vi "保存生产数据.vi"(2 "输入簇":cluster{"载具码":string, "产品码":string, "线号显示":i32}) -> (0 "error out":errorcluster caption="错误输出")   [LabVIEW 2014]
uses:
  Global.vi
  <vilib>/Utility/config.llb/Write Key (Double).vi
  <vilib>/Utility/config.llb/Write Key (String).vi
  <vilib>/Utility/config.llb/NI_LVConfig.lvlib
panel:
  out "File out":path
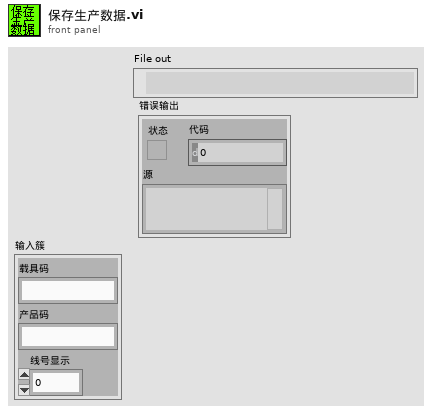
[diagram p1: front panel]
types:
  T1 = typedef "NI_LVConfig.lvlib/Config Data RefNum.ctl" = refnum<k1>
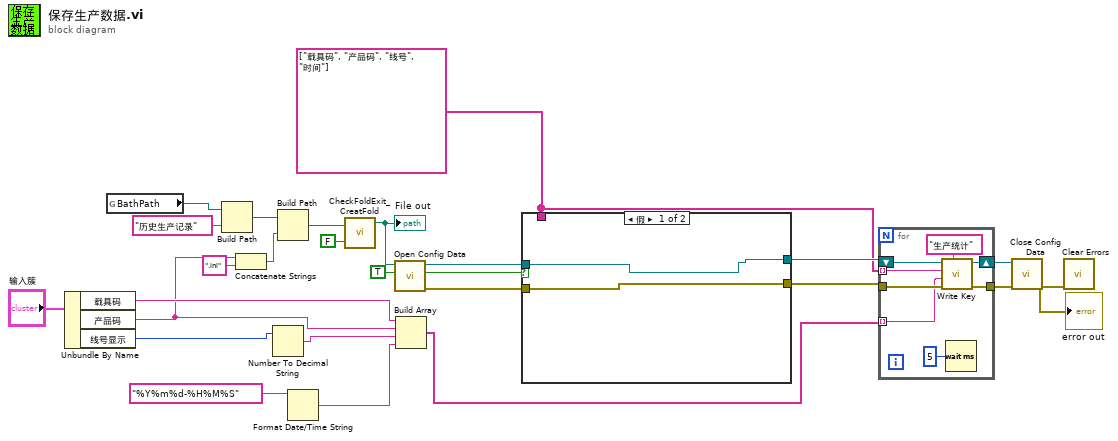
[diagram p0: block diagram]
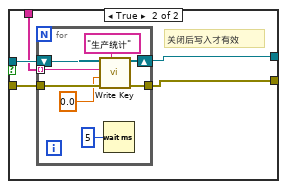
[diagram p2: hidden frame]
diagram:
  w7 = string[] ["载具码", "产品码", "线号", "时间"]
  n1 = Unbundle By Name("输入簇") -> ("载具码"=w10:string, "产品码"=w3:string, "线号显示"=w9:i32)
  n2 = global read "Global.vi" "BathPath"() -> (w21:path)
  n3 = Build Path(base path=w21, name or relative path="历史生产记录" ("名称或相对路径")) -> (appended path=w20:path)
  n4 = Concatenate Strings(w3, ".ini" ("字符串")) -> (w2:string)
  n5 = Number To Decimal String(number=w9) -> (decimal integer string=w8:string)  [unwired: 1 in]
  n6 = Build Path(base path=w20, name or relative path=w2) -> (appended path=w19:path)
  n7 = Format Date/Time String(time format string (%c)="%Y%m%d-%H%M%S") -> (date/time string=w4:string)  [unwired: 2 in]
  n8 = call "CheckFoldExit_CreatFold.vi"("path in"=w19, "FoldOrFile¡H"=FALSE) -> ("File out"=w22:path)  [unwired: 2 out]
  "File out" <- w22
  n9 = call <vilib>:"Open Config Data.vi"("create file if necessary (T)"=TRUE, "configuration file path"=w22) -> ("error out"=w24:errorcluster, "file created?"=w18:bool, "refnum"=w26:T1)  [unwired: 7 in]
  n10 = Build Array(w10, w3, w8, w4) -> (w12:string[])
  n11 = case shown="假" w18 {
    tunnel: w26 -> [w28 w33]
    tunnel: w24 -> [w27 w32]
    tunnel: w7 -> [_ w31]
    tunnel: [w28 w30] -> w16
    tunnel: [w27 w29] -> w15
    frame False {
    }
    frame True {
      # "关闭后写入才有效"
      n12 = for {
        tunnel: w31 -> [w40] mode=indexing
        shift-right: [w38] -> w30
        shift-left: w33 -> [w38]
        tunnel: w32 -> [w36]
        tunnel: [w35] -> w29
        n13 = call-poly <vilib>:"Write Key.vi"("section"="生产统计", "error in (no error)"=w36, "value"=0.0, "key"=w40, "refnum"=w38) -> ("error out"=w35:errorcluster)  [unwired: 4 in, 2 out]
        n14 = Wait (ms)(milliseconds to wait=u32 5 ("等待时间（毫秒）")) -> ()  [unwired: 1 out]
      }
    }
  }
  n15 = for {
    tunnel: w7 -> [w47] mode=indexing
    shift-right: [w45] -> w14
    shift-left: w16 -> [w45]
    tunnel: w15 -> [w43]
    tunnel: [w42] -> w13
    tunnel: w12 -> [w41] mode=indexing
    n16 = call-poly <vilib>:"Write Key.vi"("section"="生产统计", "error in (no error)"=w43, "value"=w41, "key"=w47, "refnum"=w45) -> ("error out"=w42:errorcluster)  [unwired: 4 in, 2 out]
    n17 = Wait (ms)(milliseconds to wait=u32 5 ("等待时间（毫秒）")) -> ()  [unwired: 1 out]
  }
  n18 = call <vilib>:"Close Config Data.vi"("error in (no error)"=w13, "refnum"=w14) -> ("error out"=w17:errorcluster)  [unwired: 8 in, 1 out]
  "error out" <- w17
  n19 = call <vilib>:"Clear Errors.vi"("error in (no error)"=w17) -> ()  [unwired: 5 in, 2 out]
